vi "Setting Potenza assorbita dal carico.vi"(7 "error in (no error)":errorcluster, 9 "POWER [WATT]":i32=100, 10 "VISA resource name":refnum<visa-resource-name>) -> (0 "error out":errorcluster, 3 "VISA resource name out":refnum<visa-resource-name>)   [LabVIEW 2018]
panel:
  out "resulting string":string
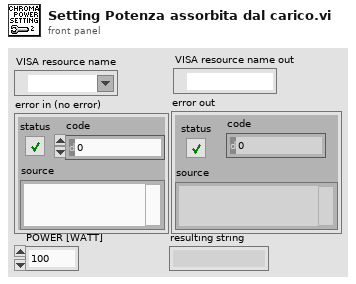
[diagram p1: front panel]
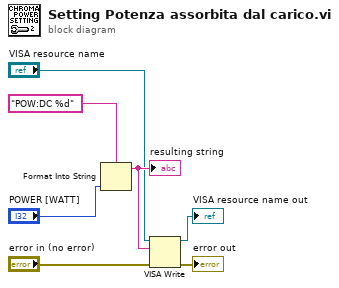
[diagram p0: block diagram]
diagram:
  n1 = Format Into String(format string="POW:DC %d", "POWER [WATT]") -> (resulting string=w5:string)  [unwired: 2 in, 1 out]
  "resulting string" <- w5
  n2 = VISA Write(VISA resource name="VISA resource name", write buffer=w5, error in (no error)="error in (no error)") -> (VISA resource name out=→"VISA resource name out":refnum<visa-resource-name>, error out=→"error out":errorcluster)  [unwired: 1 out]
